vi "7.1-6.7.1-Act UDP Server.vi"() -> ()   [LabVIEW 2010]
doc: "UDP Mutlicast Addressing Scheme:\n\n3.7 - Multicast Address: 224.0.3.7\n3.1-4.7.1 Port: 31471\n3.2-4.7.2 Port: 32472\n3.3-4.7.3 Port: 33473\n3.4-4.7.4 Port: 34474\n\n5.7 - Multicast Address: 224.0.5.7\n5.1-4.7.1 Port: 51471\n5.2-4.7.2 Port: 52472\n5.3-4.7.3 Port: 53473\n5.4-4.7.4 Port: 54474\n\n5.1-6.7.1 Port: 51671\n5.2-6.7.2 Port: 52672\n5.3-6.7.3 Port: 53673\n5.4-6.7.4 Port: 54674\n\n7.7 - Multicast Address: 224.0.7.7\n7.1-6.7.1 Port: 61671\n7.2-6.7.2 Port: 62672\n7.3-6.7.3 Port: 63673\n7.4-6.7.4 Port: 64674"
uses:
  4-High Neurons/4.0-Timing Badass.ctl
  <vilib>/Utility/tcp.llb/UDP Multicast Write-Only Open.vi
  7.0-Global.vi
panel:
  out "Super Heart Beat 2":T1
  out "Error":errorcluster
  in  "stop":bool
  out "Processed":string
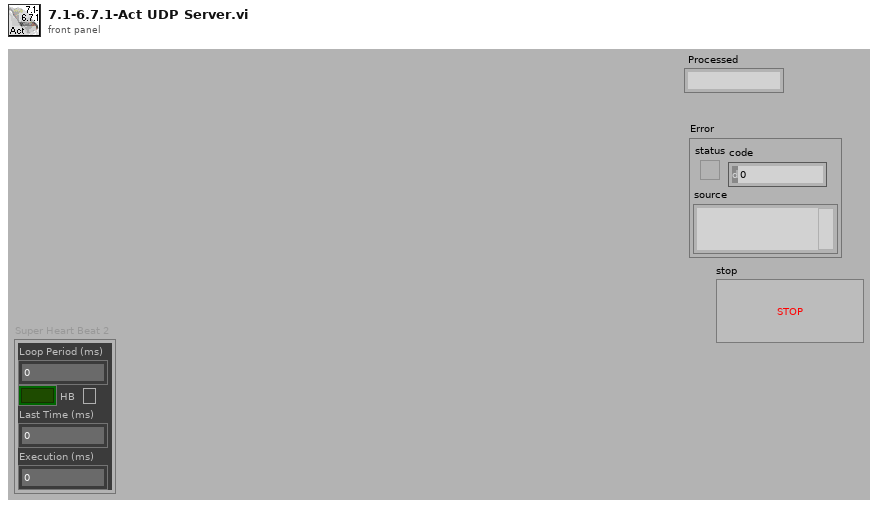
[diagram p1: front panel]
types:
  T1 = typedef "4.0-Timing Badass.ctl" = cluster{"Loop Period (ms)":u32, "HB":bool, "Last Time (ms)":u32, "Execution (ms)":u32}
  T2 = typedef "6.1-Act.ctl" = cluster{"6.1-Saitek Controller":T3, "Joystick Mode":bool, "Shutdown":bool, "Reset":bool, "Begin":bool}
  T3 = typedef "6.1-UDP Saitek.ctl" = cluster{"Trig":bool, "2":bool, "3":bool, "4":bool, "5":bool, "6":bool, "7":bool, "8":bool, "9":bool, "10":bool, "11":bool, "Pitch":i32, "Ang":bool[], "Wheel":dbl, "Roll":i32, "Yaw":i32, "Left":i32, "Right":i32}
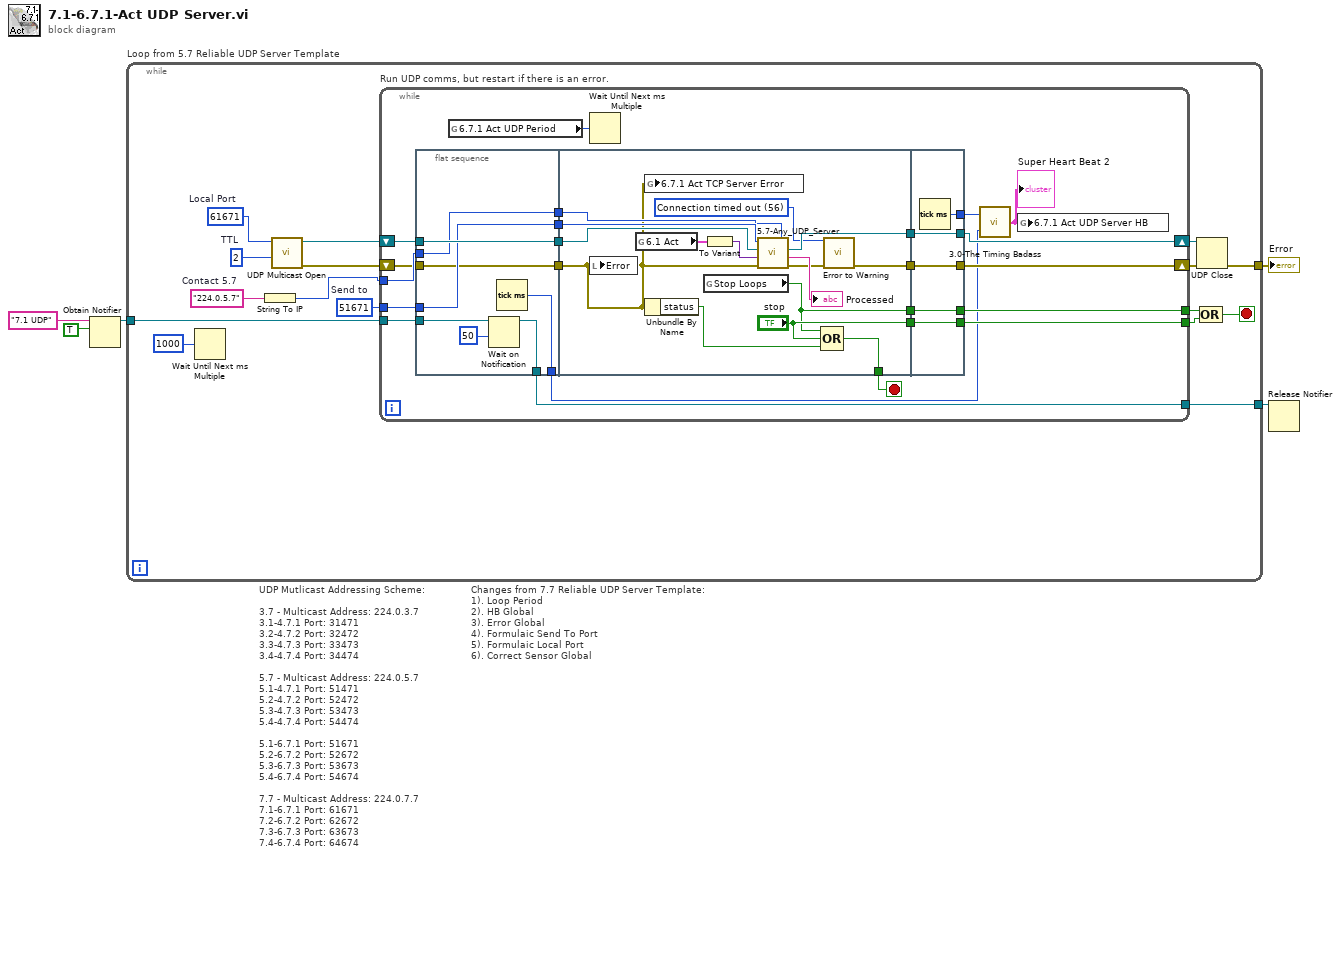
[diagram p0: block diagram]
diagram:
  # "Changes from 7.7 Reliable UDP Server Template:\n1). Loop Period\n2). HB Global\n3). Error Global\n4). Formulaic Send To Port\n5). Formulaic Local Port\n6). Correct Sensor Global"
  # "UDP Mutlicast Addressing Scheme:\n\n3.7 - Multicast Address: 224.0.3.7\n3.1-4.7.1 Port: 31471\n3.2-4.7.2 Port: 32472\n3.3-4.7.3 Port: 33473\n3.4-4.7.4 Port: 34474\n\n5.7 - Multicast Address: 224.0.5.7\n5.1-4.7.1 Port: 51471\n5.2-4.7.2 Port: 52472\n5.3-4.7.3 Port: 53473\n5.4-4.7.4 Port: 54474\n\n5.1-6.7.1 Port: 51671\n5.2-6.7.2 Port: 52672\n5.3-6.7.3 Port: 53673\n5.4-6.7.4 Port: 54674\n\n7.7 - Multicast Address: 224.0.7.7\n7.1-6.7.1 Port: 61671\n7.2-6.7.2 Port: 62672\n7.3-6.7.3 Port: 63673\n7.4-6.7.4 Port: 64674"
  n1 = Obtain Notifier(name (unnamed)="7.1 UDP", notification data type=TRUE) -> (notifier out=w3:refnum<notifier>)  [unwired: 2 in, 2 out]
  n2 = while "Loop from 5.7 Reliable UDP Server Template" {
    tunnel: [w16] -> w5
    tunnel: w3 -> [w7]
    tunnel: [w6] -> w2
    stop <- w19 stop-if-true
    w8 = "224.0.5.7"  # Contact 5.7
    w10 = u16 51671  # Send to
    w13 = u16 2  # TTL
    w14 = u16 61671  # Local Port
    n3 = Wait Until Next ms Multiple(millisecond multiple=u32 1000) -> ()  [unwired: 1 out]
    n4 = String To IP(1:w8) -> (0:w9:u32)
    n5 = call-poly <vilib>:"UDP Multicast Open.vi"("time-to-live (1)"=w13, "port"=w14) -> ("error out"=w11:errorcluster, "connection ID"=w12:refnum<k16>)  [unwired: 8 in]
    n6 = while "Run UDP comms, but restart if there is an error." {
      tunnel: [w37] -> w21
      tunnel: [w43] -> w20
      shift-right: [w41] -> w18
      shift-left: w12 -> [w42]
      shift-right: [w38] -> w17
      shift-left: w11 -> [w36]
      tunnel: w10 -> [w40]
      tunnel: w9 -> [w39]
      tunnel: w7 -> [w24]
      tunnel: [w23] -> w6
      stop <- w44 stop-if-true
      n7 = flat-sequence {
        tunnel: w36 -> [w49]
        tunnel: w39 -> [w50]
        tunnel: w40 -> [w51]
        tunnel: w42 -> [w52]
        tunnel: [w52] -> w31
        tunnel: [w51] -> w30
        tunnel: [w50] -> w29
        tunnel: [w49] -> w28
        tunnel: [w48] -> w27
        tunnel: w24 -> [w47]
        tunnel: [w46] -> w23
        tunnel: [w67] -> w44
        tunnel: ["stop"] -> w35
        tunnel: [w60] -> w34
        tunnel: [w55] -> w33
        tunnel: [w54] -> w32
        tunnel: w31 -> [w61]
        tunnel: w30 -> [w59]
        tunnel: w29 -> [w58]
        tunnel: w28 -> [w53]
        tunnel: [w69] -> w37
        tunnel: [w70] -> w38
        tunnel: [w71] -> w41
        tunnel: [w72] -> w43
        tunnel: w35 -> [w72]
        tunnel: w34 -> [w71]
        tunnel: w33 -> [w70]
        tunnel: w32 -> [w69]
        tunnel: [w68] -> w26
        frame #0 {
          n8 = Wait on Notification(notifier=w47, timeout in ms (-1)=50) -> (notifier out=w46:refnum<notifier>)  [unwired: 2 in, 3 out]
          n9 = Tick Count (ms)() -> (millisecond timer value=w48:u32)
        }
        frame #1 {
          w56 = 56 items=["No Error", "Argument Error", "Memory Full", "Out of Zone", "End of File", "File Already Open", "Generic File IO Error", "File Not Found", "File Permission Error", "Disk Full", "Duplicate Path", "Too Many Files Open", "Not Enabled", "Resource File Not Found", "Cannot Add Resource", "Resource Not Found", "Image Not Found", "Image Memory Error", "Pen Does Not Exist", "Config Bad Type", "Config Token Not Found", "Config Parse Error", "Config Memory Error", "Bad External Code Format", "Bad External Code Offset", "External Code Not Present", "Null Window", "Destroy Window Mixup", "Null Menu", "Print Aborted", "Bad Print Record", "Print Driver Error", "Windows Error During Print", "Memory Error During Print", "Print Dialog Error", "Generic Print Error", "Invalid Device Refnum", "Device Not Found", "Device Parameter Error", "Device Unit Error", "Can't Open Device", "Device Call Aborted", "Generic Error", "Cancelled By User", "Object ID Too Low", "Object ID Too High", "Object Not In Heap", "Unknown Heap", "Bad DefProc ID", "DefProc Not In Table", "Message Out Of Range", "Null Method", "Unknown Message", "Manager Call Not Supported", "Bad address", "Connection In progress", "Connection timed out", "Connection is already in progress", "Network attribute not supported", "Network error", "Address in use", "System out of memory", "Connection aborted", "Connection refused", "Connection is not connected", "Connection is already connected", "Connection closed", "Initialize error (interapplication manager)", "Bad occurrence", "Wait on unbound occurrence handler", "Occurrence queue overflow", "Bad path", "Semaphore not signaled", "Unrecognized type (interapplication manager)"] ("1st Error to Convert")
          n10 = local write "Error"(w53) -> ()
          n11 = global read "7.0-Global.vi" "6.1 Act"() -> (w63:T2)
          n12 = global write "7.0-Global.vi" "6.7.1 Act TCP Server Error"(w53) -> ()
          n13 = Unbundle By Name(w53) -> ("status"=w65:bool)
          n14 = global read "7.0-Global.vi" "Stop Loops"() -> (w54:bool)
          n15 = To Variant(anything=w63) -> (Variant=w64:variant)
          n16 = call "5.7-Any_UDP_Server.vi"("Multicast Address"=w58, "error In"=w53, "Data in"=w64, "Connection ID"=w61, "Send To Port"=w59) -> ("warning out"=w57:errorcluster, "Processed"=→"Processed":string, "Connection ID out"=w60:refnum<k16>)
          n17 = Compound Arithmetic op=OR(w54, "stop", w65) -> (w67:bool)
          n18 = call <vilib>:"Error to Warning.vi"("1st Error to Convert"=w56, "error in"=w57) -> ("warning out"=w55:errorcluster)  [unwired: 13 in]
        }
        frame #2 {
          n19 = Tick Count (ms)() -> (millisecond timer value=w68:u32)
        }
      }
      n20 = global read "7.0-Global.vi" "6.7.1 Act UDP Period"() -> (w22:u32)
      n21 = Wait Until Next ms Multiple(millisecond multiple=w22) -> ()  [unwired: 1 out]
      n22 = call "3.0-The Timing Badass.vi"("Start"=w27, "End"=w26) -> ("Super Heart Beat"=w25:T1)
      "Super Heart Beat 2" <- w25
      n23 = global write "7.0-Global.vi" "6.7.1 Act UDP Server HB"(w25) -> ()
    }
    n24 = UDP Close(connection ID=w18, 8:w17) -> (error out=w16:errorcluster)  [unwired: 1 out]
    n25 = Compound Arithmetic op=OR(w21, w20) -> (w19:bool)
  }
  "Error" <- w5
  n26 = Release Notifier(notifier=w2) -> ()  [unwired: 2 in, 3 out]
